vi "simple.vi"() -> (3 "Numeric":i32)   [LabVIEW 2012]
panel:
  out "error out":errorcluster
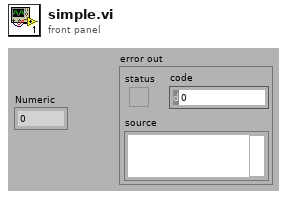
[diagram p1: front panel]
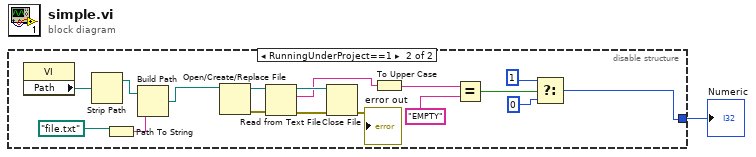
[diagram p0: block diagram]
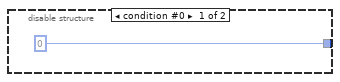
[diagram p2: hidden frame]
diagram:
  n1 = disable-structure shown="RunningUnderProject==1" {
    disable-tunnel: [0 w18] -> w1
    frame condition #0 {
    }
    frame condition #1 (active) {
      n2 = property class="VI"() -> ("Path"=w8:path)  [unwired: 2 in, 2 out]
      n3 = Strip Path(path=w8) -> (stripped path=w7:path)  [unwired: 1 out]
      n4 = Path To String(path=path "file.txt" ("Path")) -> (string=w6:string)
      n5 = Build Path(base path=w7, name or relative path=w6) -> (appended path=w4:path)
      n6 = Open/Create/Replace File(file path (use dialog)=w4) -> (refnum out=w17:refnum<file>, error out=w16:errorcluster)  [unwired: 5 in, 1 out]
      n7 = Read from Text File(file (use dialog)=w17, error in=w16) -> (refnum out=w14:refnum<file>, text=w12:string, error out=w15:errorcluster)  [unwired: 2 in, 1 out]
      n8 = Close File(refnum=w14, error in=w15) -> (error out=→"error out":errorcluster)  [unwired: 1 out]
      n9 = To Upper Case(1:w12) -> (0:w10:string)
      n10 = Equal?(x=w10, y="EMPTY") -> (x = y?=w11:bool)
      n11 = Select(t=1 ("Numeric"), s=w11, f=0 ("y")) -> (s? t:f=w18:i32)
    }
  }
  "Numeric" <- w1
